vi "Create Filter from Transfer Function.vi"() -> ()   [LabVIEW 2023]
doc: "Demonstrates how to use the DFD Build Filter from Transfer Function VI to create a filter from a transfer function. This VI provides some example transfer functions to show the default structure of the new filter.\n\nComplete the following steps to use this VI.\n1) Run the VI.\n2) Select an example transfer function.\n3) Observe the magnitude response of the created filter.\n4) Observe the default filter structure of the created filter.\n5) View the corresponding transfer function, including the numerator and denominator, on the User Defined page.\n6) Change the elements of the numerator or denominator or add more elements.\n7) Observe the magnitude response.\n8) Click the <B>STOP</B> button to stop this VI."
uses:
  <vilib>/addons/Digital Filter Design/Analysis.llb/DFD Plot Freq Response (Linear-Spaced).vi
  <vilib>/addons/Digital Filter Design/NI_DigFilterLicensed.lvlib
panel:
  out "Error Message":string
  in  "stop":bool
  in  "Tab Control":enum32{"Examples", "User Defined"}(tab)
  in  "Options":i32(listbox)
  in  "Denominator":dbl[](array[numeric])=[1.0]
  in  "Numerator":dbl[](array[numeric])=[1.0]
  out "Magnitude Response":cluster{"f0":dbl, "df":dbl, "magnitude":dbl[]}[](graph)
  out "Default Filter Structure":u16(ring) items=["Invalid", "FIR Direct Form", "FIR Direct Form Transposed", "FIR Symmetric", "FIR Antisymmetric", "IIR Direct Form I", "IIR Direct Form I Transposed", "IIR Direct Form II", "IIR Direct Form II Transposed", "IIR Cascaded Second-Order Sections Form I", "IIR Cascaded Second-Order Sections Form I Transposed", "IIR Cascaded Second-Order Sections Form II", "IIR Cascaded Second-Order Sections Form II Transposed", "Lattice Allpass (basic sections)", "Lattice Allpass (one multiplier sections)", "Lattice Allpass (normalized sections)", "Lattice AR (basic sections)", "Lattice AR (one multiplier sections)", "Lattice AR (normalized sections)", "Lattice MA (minimum phase)", "Lattice MA (maximum phase)", "Lattice ARMA (basic sections)", "Lattice ARMA (one multiplier sections)", "Lattice ARMA (normalized sections)"]
  # "Select Help>>Show Context Help and move the cursor over the VI icon for more information."
  # "Select an example from the list above and obtain\nthe corresponding numerator and denominator\nvalues on the User Defined page."
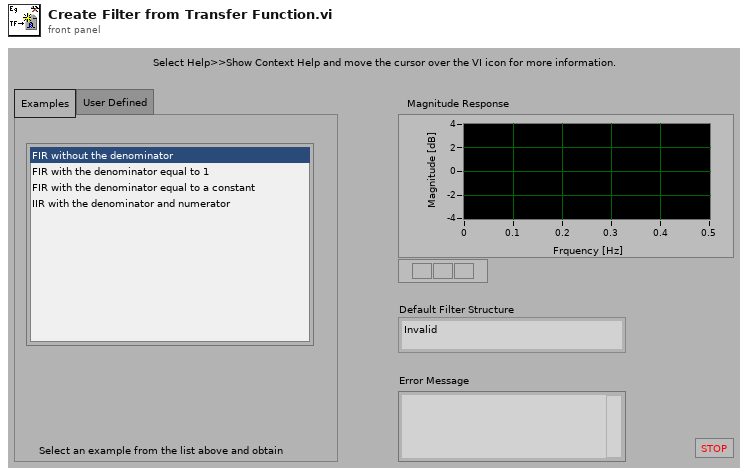
[diagram p1: front panel]
types:
  T1 = typedef "NI_DigFilterLicensed.lvlib/DFD Filter Obj.ctl" = cluster{"mSRate_Fs":dbl, "mSRate_Version":string, "mSRate_Comments":string, "mSRate_OrgCoef":T2, "mSRate_CurCoef":T2, "mSRate_Quantized?":bool, "mSRate_QCoef":T2, "mSRate_QSettings":T4[], "mSRate_Order":i32, "mSRate_Scaling":cluster{"mSRate_ScaleByPowerOf2?":bool, "mSRate_ScaleType":T6}}
  T2 = typedef "NI_DigFilterLicensed.lvlib/DFD Filter Coef.ctl" = cluster{"type":T3, "gain":dbl, "coef a (k)":dbl[], "coef b (v)":dbl[]}
  T3 = typedef "NI_DigFilterLicensed.lvlib/DFD Filter Structure Type Selector.ctl" = enum16{"Undefined", "FIR Direct Form", "FIR Direct Form Transposed", "FIR Symmetric", "FIR Antisymmetric", "IIR Direct Form I", "IIR Direct Form I Transposed", "IIR Direct Form II", "IIR Direct Form II Transposed", "IIR Cascaded Second Order Sections Form I", "IIR Cascaded Second Order Sections Form I Transposed", "IIR Cascaded Second Order Sections Form II", "IIR Cascaded Second Order Sections Form II Transposed", "Lattice Allpass (basic sections)", "Lattice Allpass (one multiplier sections)", "Lattice Allpass (normalized sections)", "Lattice AR (basic sections)", "Lattice AR (one multiplier sections)", "Lattice AR (normalized sections)", "Lattice MA (minimum phase)", "Lattice MA (maximum phase)", "Lattice ARMA (basic sections)", "Lattice ARMA (one multiplier sections)", "Lattice ARMA (normalized sections)"}
  T4 = typedef "NI_DigFilterLicensed.lvlib/dfd_Internal Quantization Settings.ctl" = cluster{"source":T5, "wl":i16, "iwl":i16, "overflow mode":enum16{"Saturation", "Wrap"}, "rounding mode":enum16{"Nearest", "Truncation"}, "signed?":bool}
  T5 = typedef "NI_DigFilterLicensed.lvlib/dfd_Internal Quantization Srcs.ctl" = u16
  T6 = typedef "NI_DigFilterLicensed.lvlib/DFD Coef Norm Type.ctl" = enum16{"No Norm", "Time Domain 1-Norm", "Time Domain 2-Norm", "Time Domain Inf-Norm"}
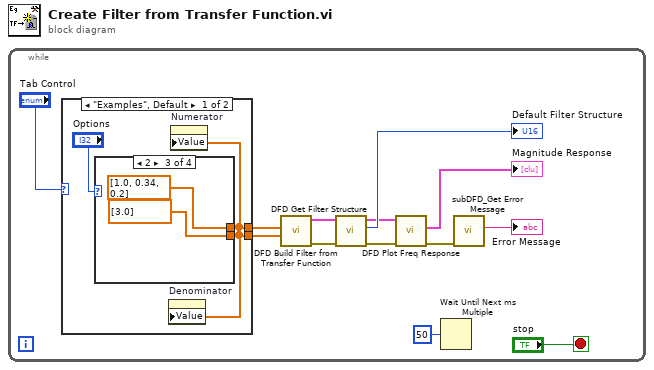
[diagram p0: block diagram]
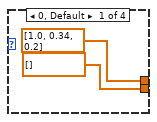
[diagram p2: hidden frame]
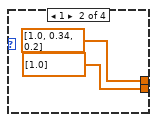
[diagram p3: hidden frame]
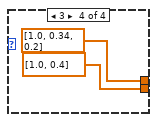
[diagram p4: hidden frame]
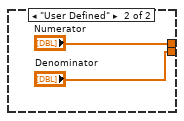
[diagram p5: hidden frame]
diagram:
  n1 = while {
    stop <- "stop" stop-if-true
    n2 = case shown="\"Examples\", Default" "Tab Control" {
      tunnel: [w15 "Numerator"] -> w13
      tunnel: [w14 "Denominator"] -> w12
      frame "Examples", Default {
        n3 = case shown="2" "Options" {
          tunnel: [dbl[] [1.0, 0.34, 0.2] dbl[] [1.0, 0.34, 0.2] dbl[] [1.0, 0.34, 0.2] dbl[] [1.0, 0.34, 0.2]] -> w15
          tunnel: [dbl[] [] dbl[] [1.0] dbl[] [3.0] dbl[] [1.0, 0.4]] -> w14
          frame 0, Default {
          }
          frame 1 {
          }
          frame 2 {
          }
          frame 3 {
          }
        }
        n4 = property on="Denominator" class="Arr (strict)"("Value"=w14) -> ()  [unwired: 2 in, 2 out]
        n5 = property on="Numerator" class="Arr (strict)"("Value"=w15) -> ()  [unwired: 2 in, 2 out]
      }
      frame "User Defined" {
      }
    }
    n6 = call <vilib>:"DFD Build Filter from Transfer Function.vi"("denominator"=w12, "numerator"=w13) -> ("error out"=w11:errorcluster, "filter out"=w9:T1)  [unwired: 3 in, 5 out]
    n7 = call <vilib>:"DFD Get Filter Structure.vi"("error in (no error)"=w11, "filter in"=w9) -> ("error out"=w8:errorcluster, "structure"=→"Default Filter Structure":u16, "filter out"=w3:T1)  [unwired: 7 out]
    n8 = call-poly <vilib>:"DFD Plot Freq Response.vi"("error in (no error)"=w8, "filter in"=w3) -> ("error out"=w2:errorcluster, "magnitude response"=→"Magnitude Response":cluster{"f0":dbl, "df":dbl, "values":dbl[]}[])  [unwired: 6 in, 2 out]
    n9 = Wait Until Next ms Multiple(millisecond multiple=u32 50) -> ()  [unwired: 1 out]
    n10 = call <vilib>:"subDFD_Get Error Message.vi"("error in (no error)"=w2) -> ("Error Message"=→"Error Message":string)  [unwired: 10 out]
  }
